vi "RemoveObject.vi"(1 "remote ref":refnum<class "G#Object.lvclass">, 5 "error in (no error)":errorcluster) -> (15 "proxy ref":refnum<class "G#RemoteProxy.lvclass">, 19 "error out":errorcluster)   [LabVIEW 2017, in "G#RemoteProxy.lvclass"]
doc: "Removes a cached object."
uses:
  <vilib>/addons/_AddQ/G#Debugger/G#RemoteProxy/G#RemoteProxy.lvclass
  <vilib>/addons/_AddQ/G#Object/G#Object.lvclass
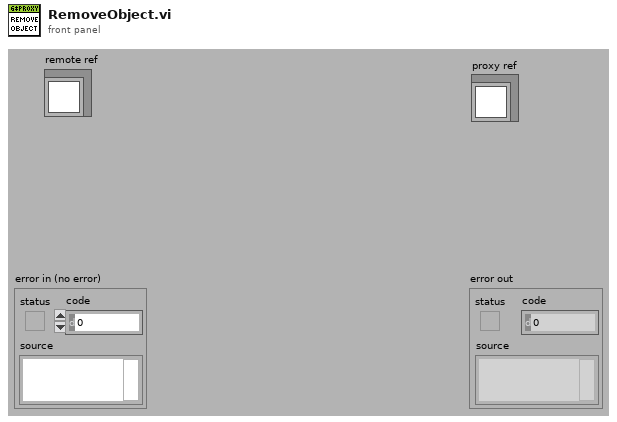
[diagram p1: front panel]
types:
  T1 = typedef "G#RemoteProxy.lvclass/ClassAttributesRef.ctl" = refnum<data-value>
  T2 = typedef "G#RemoteProxy.lvclass/ClassAttributesProxy.ctl" = cluster{"NoActiveProject":bool, "FullClassNames":string[], "FullClassPaths":path[], "RemoteRefs":refnum<class "G#Object.lvclass">[], "ProxyRefs":refnum<class "G#RemoteProxy.lvclass">[], "RemoteClassName":string[], "ProxyClassRefs":refnum<class "G#RemoteProxy.lvclass">[]}
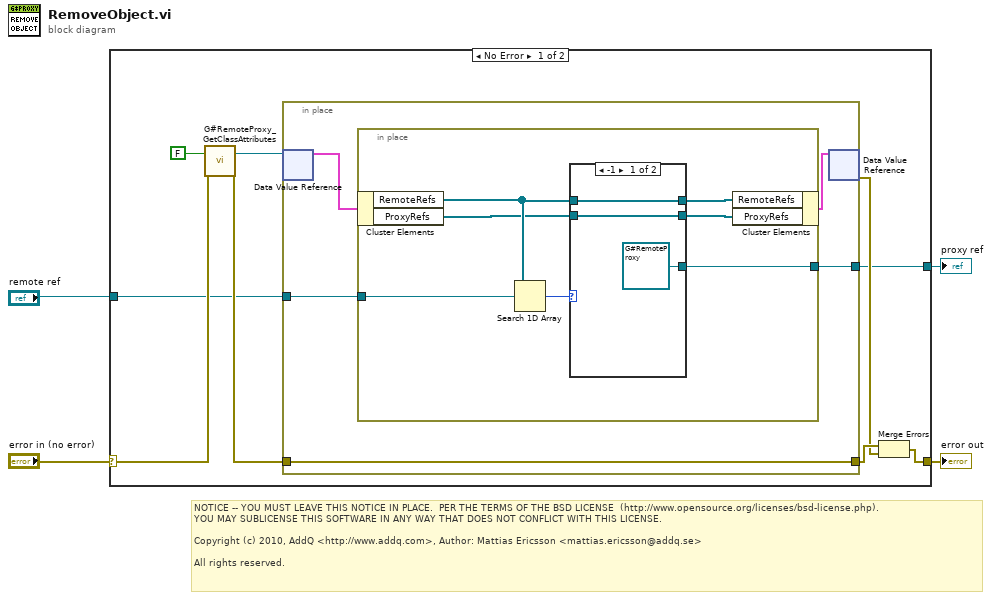
[diagram p0: block diagram]
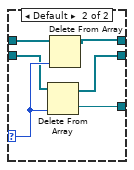
[diagram p2: hidden frame]
diagram:
  # "NOTICE -- YOU MUST LEAVE THIS NOTICE IN PLACE.  PER THE TERMS OF THE BSD LICENSE  (http://www.opensource.org/licenses/bsd-license.php).\nYOU MAY SUBLICENSE THIS SOFTWARE IN ANY WAY THAT DOES NOT CONFLICT WITH THIS LICENSE.\n\nCopyright (c) 2010, AddQ <http://www.addq.com>, Author: Mattias Ericsson <mattias.ericsson@addq.se>\n\nAll rights reserved."
  n1 = case shown="No Error" "error in (no error)" {
    selector: "error in (no error)" -> [w13 w35]
    tunnel: [w10 w35] -> w3
    tunnel: "remote ref" -> [w6 _]
    tunnel: [w5 _] -> w1
    frame No Error {
      n2 = call <vilib>:"G#RemoteProxy_GetClassAttributes.vi"("return data? (T)"=FALSE ("return data"), "error in (no error)"=w13) -> ("class attributes ref"=w11:T1, "error out"=w12:errorcluster)  [unwired: 14 in, 2 out]
      n3 = in-place {
        in-place-border: w12 -> [w16]
        in-place-border: [w16] -> w8
        in-place-border: w6 -> [w15]
        in-place-border: [w14] -> w5
        n4 = in-place-dvr #1(w11) -> (w17:T2)  [unwired: 1 out]
        n5 = in-place {
          in-place-border: w15 -> [w25]
          in-place-border: [w19] -> w14
          n6 = in-place-cluster #2(w17) -> ("RemoteRefs"=w23:refnum<class "G#Object.lvclass">[], "ProxyRefs"=w21:refnum<class "G#RemoteProxy.lvclass">[])
          n7 = Search 1D Array(1D array=w23, element=w25) -> (index of element=w24:i32)  [unwired: 1 in]
          n8 = case shown="-1" w24 {
            selector: w24 -> [_ w32]
            tunnel: w23 -> [w28 w34]
            tunnel: [w28 w33] -> w22
            tunnel: w21 -> [w27 w31]
            tunnel: [w27 w30] -> w20
            tunnel: [refnum<class "G#RemoteProxy.lvclass"> refnum ("G#RemoteProxy.lvclass") w29] -> w19
            frame -1 {
            }
            frame Default {
              n9 = Delete From Array(array=w31, index=w32) -> (deleted portion=w29:refnum<class "G#RemoteProxy.lvclass">, array with subset deleted=w30:refnum<class "G#RemoteProxy.lvclass">[])  [unwired: 1 in]
              n10 = Delete From Array(array=w34, index=w32) -> (array with subset deleted=w33:refnum<class "G#Object.lvclass">[])  [unwired: 1 in, 1 out]
            }
          }
          n11 = in-place-cluster #2("RemoteRefs"=w22, "ProxyRefs"=w20) -> (w18:T2)
        }
        n12 = in-place-dvr #1(w18) -> (w7:errorcluster)  [unwired: 1 out]
      }
      n13 = Merge Errors(w8, w7) -> (w10:errorcluster)
    }
    frame Error {
    }
  }
  "error out" <- w3
  "proxy ref" <- w1
